vi "test_CCDSetAndGetExposureTime.vi"(6 "Delay between send and receive [ms]":i32=100, 7 "Test should pass":bool=TRUE, 8 "error in":errorcluster, 9 "tear down connection":bool=TRUE, 10 "set-up a connection":bool=TRUE, 11 "device selection":enum16{"monochromator", "CCD", "SCD"}(ring)=enum."CCD") -> (0 "error out":errorcluster)   [LabVIEW 2023]
uses:
  Classes/CCD/CCD.lvclass
  <vilib>/addons/_JKI Toolkits/Caraya/classes/Assert/Assert Equal Value and Type_Variant.vi
  <vilib>/addons/_JKI Toolkits/Caraya/classes/Assert/Assert Not Error.vi
  <vilib>/addons/_JKI Toolkits/Caraya/classes/Test/Test.lvclass
  <vilib>/addons/_JKI Toolkits/Caraya/classes/Assert/Assert.lvclass
panel:
  # "Connector Pane"
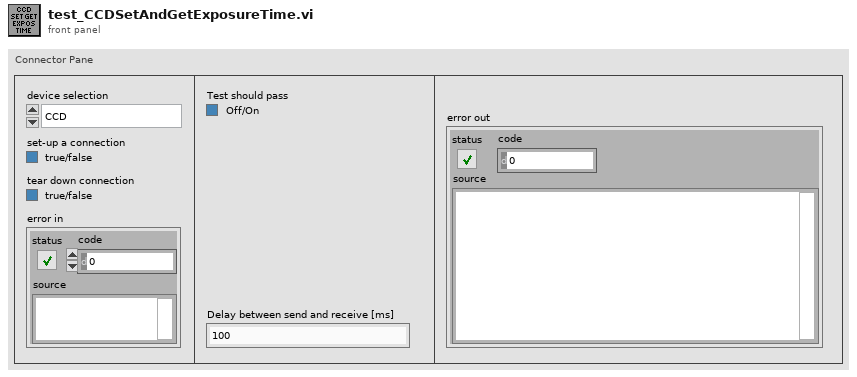
[diagram p1: front panel]
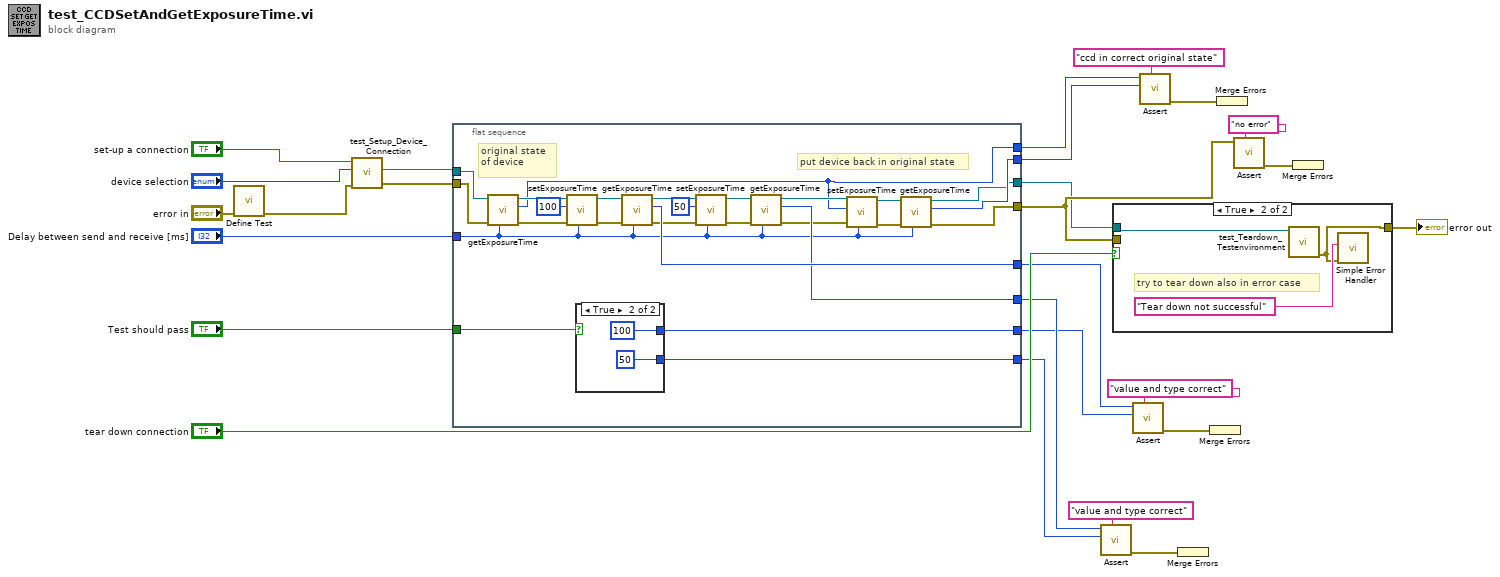
[diagram p0: block diagram]
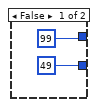
[diagram p2: hidden frame]
diagram:
  n1 = call <vilib>:"Define Test.vi"("error in (no error)"="error in") -> ("error out"=w2:errorcluster)  [unwired: 9 in, 1 out]
  n2 = call "test_Setup_Device_Connection.vi"("error in (no error)"=w2, "device selection"="device selection", "set-up a connection"="set-up a connection") -> ("error out"=w3:errorcluster, "CCD.lvclass"=w4:refnum<class "CCD.lvclass">)  [unwired: 5 in, 2 out]
  n3 = flat-sequence {
    tunnel: w3 -> [w48]
    tunnel: w4 -> [w49]
    tunnel: [w28] -> w17
    tunnel: "Test should pass" -> [w52]
    tunnel: [w29] -> w16
    tunnel: [w36] -> w15
    tunnel: [w51] -> w14
    tunnel: [w42] -> w13
    tunnel: [w50] -> w12
    tunnel: [w31] -> w9
    tunnel: [w30] -> w8
    tunnel: "Delay between send and receive [ms]" -> [w27]
    frame #0 {
      # "put device back in original state"
      # "original state of device"
      n4 = call "getExposureTime.vi"("Delay between send and receive [ms]"=w27, "error in (no error)"=w48, "CCD in"=w49) -> ("error out"=w46:errorcluster, "time [ms] or [us]"=w31:i32, "CCD out"=w47:refnum<class "CCD.lvclass">)  [unwired: 6 in]
      n5 = call "setExposureTime.vi"("Delay between send and receive [ms]"=w27, "error in (no error)"=w46, "exposure time [ms] or [us]"=100 ("exposure time [ms]"), "CCD in"=w47) -> ("error out"=w44:errorcluster, "CCD out"=w43:refnum<class "CCD.lvclass">)  [unwired: 4 in, 2 out]
      n6 = case shown="True" w52 {
        tunnel: [49 ("exposure time [ms]") 50 ("exposure time [ms]")] -> w51
        tunnel: [99 ("exposure time [ms]") 100 ("exposure time [ms]")] -> w50
        frame False {
        }
        frame True {
        }
      }
      n7 = call "getExposureTime.vi"("Delay between send and receive [ms]"=w27, "error in (no error)"=w44, "CCD in"=w43) -> ("error out"=w38:errorcluster, "time [ms] or [us]"=w42:i32, "CCD out"=w39:refnum<class "CCD.lvclass">)  [unwired: 6 in]
      n8 = call "setExposureTime.vi"("Delay between send and receive [ms]"=w27, "error in (no error)"=w38, "exposure time [ms] or [us]"=50 ("exposure time [ms]"), "CCD in"=w39) -> ("error out"=w41:errorcluster, "CCD out"=w40:refnum<class "CCD.lvclass">)  [unwired: 4 in, 2 out]
      n9 = call "getExposureTime.vi"("Delay between send and receive [ms]"=w27, "error in (no error)"=w41, "CCD in"=w40) -> ("error out"=w33:errorcluster, "time [ms] or [us]"=w36:i32, "CCD out"=w34:refnum<class "CCD.lvclass">)  [unwired: 6 in]
      n10 = call "setExposureTime.vi"("Delay between send and receive [ms]"=w27, "error in (no error)"=w33, "exposure time [ms] or [us]"=w31, "CCD in"=w34) -> ("error out"=w35:errorcluster, "CCD out"=w32:refnum<class "CCD.lvclass">)  [unwired: 4 in, 2 out]
      n11 = call "getExposureTime.vi"("Delay between send and receive [ms]"=w27, "error in (no error)"=w35, "CCD in"=w32) -> ("error out"=w28:errorcluster, "time [ms] or [us]"=w30:i32, "CCD out"=w29:refnum<class "CCD.lvclass">)  [unwired: 6 in]
    }
  }
  n12 = call-poly <vilib>:"Assert.vi"("Label"="value and type correct" ("Label (VI Title)"), "Y"=w14, "X"=w15) -> ("error out"=w25:errorcluster)  [unwired: 7 in, 1 out]
  n13 = case shown="True" "tear down connection" {
    tunnel: w16 -> [_ w59]
    tunnel: [w57 w58] -> w7
    tunnel: w17 -> [w57 _]
    frame False {
    }
    frame True {
      # "try to tear down also in error case"
      n14 = call "test_Teardown_Testenvironment.vi"("GenericDevice.lvclass"=w59) -> ("error out"=w58:errorcluster)  [unwired: 9 in, 1 out]
      n15 = call <vilib>:"Simple Error Handler.vi"("error source (\" \")"="Tear down not successful" ("error source (\" \")"), "error in (no error)"=w58) -> ()  [unwired: 3 in, 5 out]
    }
  }
  "error out" <- w7
  n16 = call-poly <vilib>:"Assert.vi"("Label"="value and type correct" ("Label (VI Title)"), "Y"=w12, "X"=w13) -> ("error out"=w24:errorcluster)  [unwired: 7 in, 1 out]
  n17 = call-poly <vilib>:"Assert.vi"("Label"="ccd in correct original state" ("Label (VI Title)"), "Y"=w8, "X"=w9) -> ("error out"=w11:errorcluster)  [unwired: 7 in, 1 out]
  n18 = Merge Errors(w25) -> ()  [unwired: 1 out]
  n19 = Merge Errors(w24) -> ()  [unwired: 1 out]
  n20 = Merge Errors(w11) -> ()  [unwired: 1 out]
  n21 = call-poly <vilib>:"Assert.vi"("Label"="no error" ("Label (VI Title)"), "Not Error?"=w17) -> ("error out"=w19:errorcluster)  [unwired: 8 in, 1 out]
  n22 = Merge Errors(w19) -> ()  [unwired: 1 out]
